vi "SaveDeviceHeader.vi"(0 "File Refnum in":refnum<file>, 2 "Channel Number":i32, 5 "Filename":string, 9 "Array Titles":string, 11 "error in (no error)":errorcluster, 12 "Temperature":dbl, 13 "Humidity":dbl, 14 "Strip Segment":string) -> (4 "File Refnum out":refnum<file>, 6 "Header string":string, 10 "error out":errorcluster)   [LabVIEW 2019]
uses:
  globals/QC_MeasurementSetup.vi
  globals/QC_RunInformation.vi
  <vilib>/regexp/Match Regular Expression.xnode
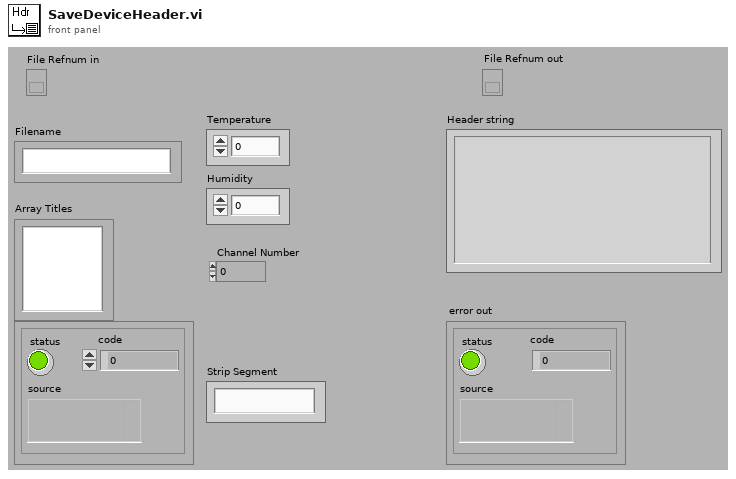
[diagram p1: front panel]
types:
  T1 = cluster{"User":string, " Institute":string, " Test Time":string, " Test Date":string, "Instruments":string, "Sensor IDS":string[], "IV Test?":bool, "CV Test? ":bool, "LCS Test? ":bool, "No. of Ch.":u16, " Current Sensor":string, " Current Test":string, "Arduino DP Map":string[], "Sensor BW":string[], "Sensor Types":string[], "Data directory":string, "7036 Channel Map":string[], "7054 1 Map":string[], "7054 2 Map ":string[], "7054 3 Map ":string[]}
  T2 = cluster{"Supply":refnum<class "SupplyControl.lvclass">, "LCR":refnum<class "LCRControl.lvclass">, "Arduino":refnum<class "ArduinoControl.lvclass">, "Switching":refnum<class "Switching.lvclass">, "SMU Name":string, " LCR Name":string, " Volt Name ":string, " Switching GPIB Address ":string, "Temperature Readout":enum16{"Read Arduino", "Enter manually"}, "Voltmeter Visa":refnum<visa-resource-name>}
  T3 = cluster{"Supply":refnum<class "SupplyControl.lvclass">, "LCR":refnum<class "LCRControl.lvclass">, "Initial Voltage [V]":dbl, "Final Voltage [V]":dbl, "Step Size [V]":dbl, "Step Interval [s]":i32, "Number Of Steps":u32, "AC frequency [Hz]":i32, "RC Configuration":u16, "AC amplitude [V]":dbl, "Ramp down steps [V]":dbl, "Ramp down Interval [s]":i32, "Set Current Limit?":bool, "Current Limit [µA]":dbl, "Temperature Readout":enum16{"Read Arduino", "Enter manually"}, "Arduino":refnum<class "ArduinoControl.lvclass">, "Supply Name":string, "LCR Name":string, "V_depletion Limit [V]":dbl, "Switching":refnum<class "Switching.lvclass">, "Matrix used?":bool, "Matrix X Channels":cluster{"Bias Supply / SMU LO":i32, "Bias Supply / SMU HI":i32, "CV Box LO":i32, "CV Box HI":i32, "CV Box LO IN":i32, "CV Box HI IN":i32, "Volt meter LO":i32, "Volt meter HI":i32, "Mux1 C1":i32, "Mux1 C2":i32, "Mux2 C1":i32, "Mux2 C2":i32}, "CV Test?":bool}
  T4 = cluster{"Bias Supply":refnum<class "SupplyControl.lvclass">, "SMU":refnum<class "SupplyControl.lvclass">, "LCR":refnum<class "LCRControl.lvclass">, "Probe Card Channels":i32, "Bias Voltage [V]":dbl, "First strip":i32, "Last strip":i32, "Base Voltage [V]":dbl, "Base Ramp Step [V]":dbl, "Base Ramp Interval [ms]":u32, "High Voltage [V]":dbl, "High Ramp Step [V]":dbl, "High Ramp Interval [ms]":u32, "AC frequency [Hz]":i32, "AC amplitude [V]":dbl, "RC Configuration":u16, "Single Needle":bool, "Temperature Readout":enum16{"Read Arduino", "Enter manually"}, "Arduino":refnum<class "ArduinoControl.lvclass">, "Fraction of good strips [%]":dbl, "ProbeStation":refnum<class "ProbeStationControl.lvclass">, "Switching":refnum<class "Switching.lvclass">, "Matrix used?":bool, "Matrix X Channels":cluster{"Bias Supply / SMU LO":i32, "Bias Supply / SMU HI":i32, "CV Box LO":i32, "CV Box HI":i32, "CV Box LO IN":i32, "CV Box HI IN":i32, "Volt meter LO":i32, "Volt meter HI":i32, "Mux1 C1":i32, "Mux1 C2":i32, "Mux2 C1":i32, "Mux2 C2":i32}, "Pinholes Y/N":bool, "Capacitance Y/N":bool, "Resistance Y/N":bool, "Bias Supply Name":string, "SMU Name":string, "LCR Name":string}
  T5 = cluster{"Sensor Serial No.:":string, "Wafer Serial No.:":string, "Batch:":string, "Manufacturer:":string, "Device Category:":string, "Database Serial No.:":string, "Date Initiated:":string, "Time Initiated:":string, "Test":string, "Instruments used:":string, "Probeplan used:":string, "End of Run comment:":string, "User:":string}
  T6 = cluster{"Supply":refnum<class "SupplyControl.lvclass">, "LCR":refnum<class "LCRControl.lvclass">, "Initial Voltage [V]":dbl, "Final Voltage [V]":dbl, "Step Size [V]":dbl, "Step Interval [s]":i32, "Number Of Steps":u32, "AC frequency [Hz]":i32, "RC Configuration":u16, "AC amplitude [V]":dbl, "Ramp down steps [V]":dbl, "Ramp down Interval [s]":i32, "Set Current Limit?":bool, "Current Limit [µA]":dbl, "Temperature Readout":enum16{"Read Arduino", "Enter manually"}, "Arduino":refnum<class "ArduinoControl.lvclass">, "Supply Name":string, "LCR Name":string, "C_is Limit [pF/cm]":dbl, "Switching":refnum<class "Switching.lvclass">, "Matrix used?":bool, "Matrix X Channels":cluster{"Bias Supply / SMU LO":i32, "Bias Supply / SMU HI":i32, "CV Box LO":i32, "CV Box HI":i32, "CV Box LO IN":i32, "CV Box HI IN":i32, "Volt meter LO":i32, "Volt meter HI":i32, "Mux1 C1":i32, "Mux1 C2":i32, "Mux2 C1":i32, "Mux2 C2":i32}}
  T7 = cluster{"Supply":refnum<class "SupplyControl.lvclass">, "Voltage [V]":dbl, "Measurement Interval [s]":i32, "Test Duration":u32, "Ramp up steps [V]":dbl, "Ramp up Interval [s]":u32, "Ramp down steps [V]":dbl, "Ramp down Interval [s]":i32, "Set Current Limit?":bool, "Current Limit [µA]":dbl, "Temperature Readout":enum16{"Read Arduino", "Enter manually"}, "Arduino":refnum<class "ArduinoControl.lvclass">, "Supply Name":string, "Maximum current fluctuation [%]":dbl, "Switching.lvclass":refnum<class "Switching.lvclass">, "Matrix used?":bool, "Matrix X Channels":cluster{"Bias Supply / SMU LO":i32, "Bias Supply / SMU HI":i32, "CV Box LO":i32, "CV Box HI":i32, "CV Box LO IN":i32, "CV Box HI IN":i32, "Volt meter LO":i32, "Volt meter HI":i32, "Mux1 C1":i32, "Mux1 C2":i32, "Mux2 C1":i32, "Mux2 C2":i32}, "LCS Test?":bool, "Number of Steps":i32, "Norm. to Temp.":dbl}
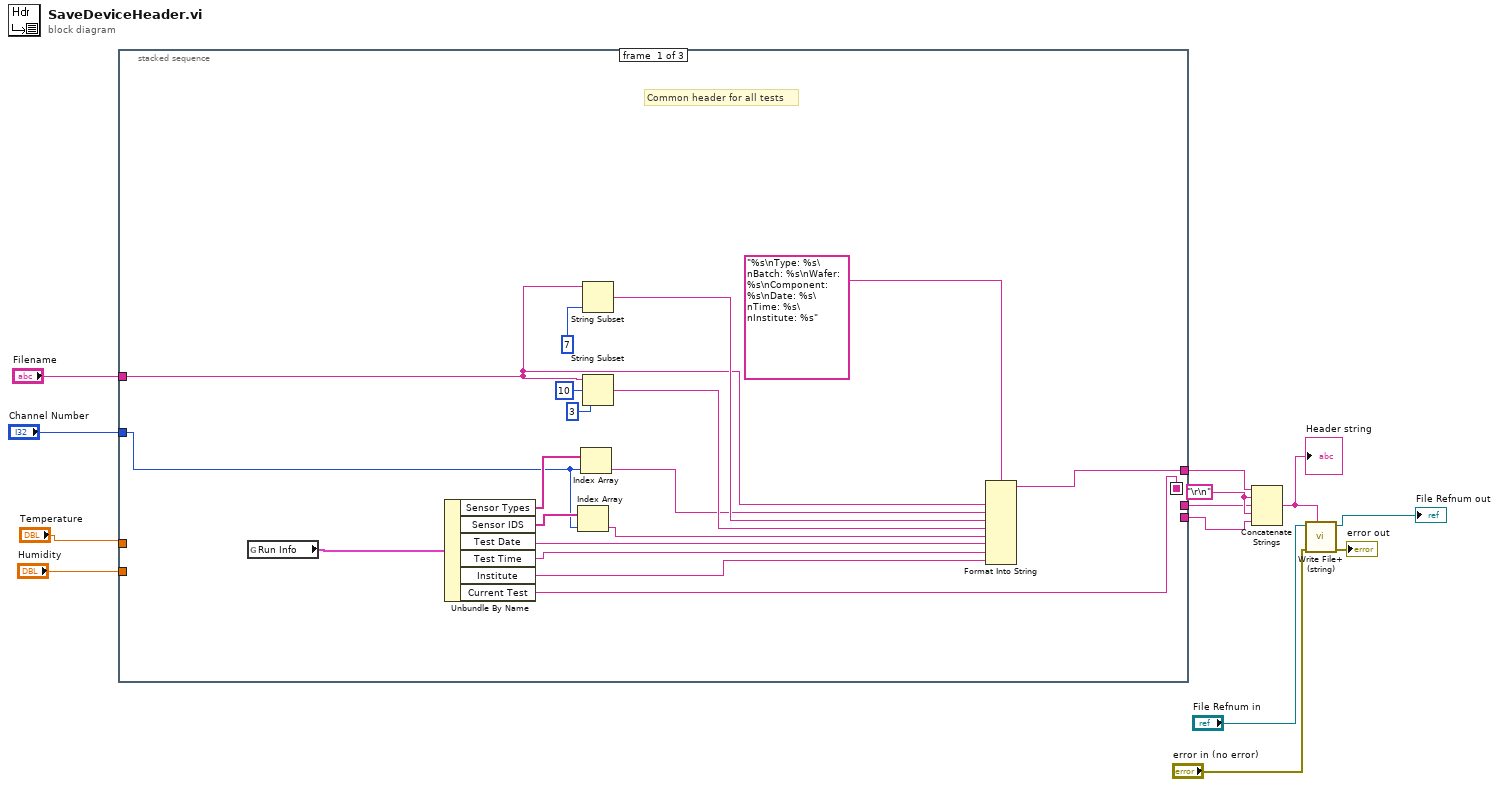
[diagram p0: block diagram]
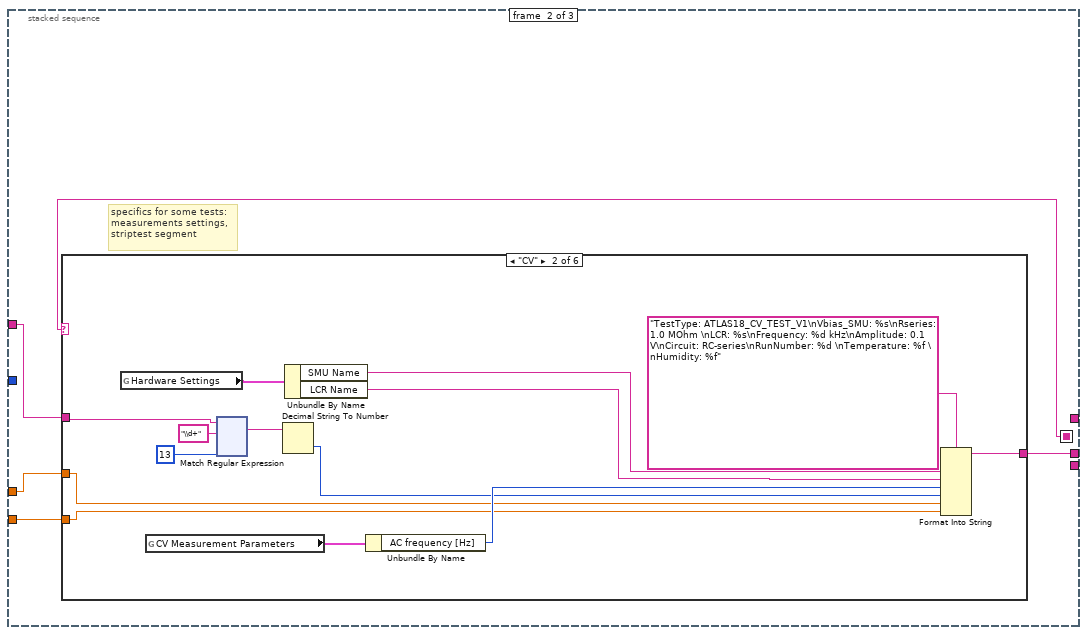
[diagram p2: hidden frame]
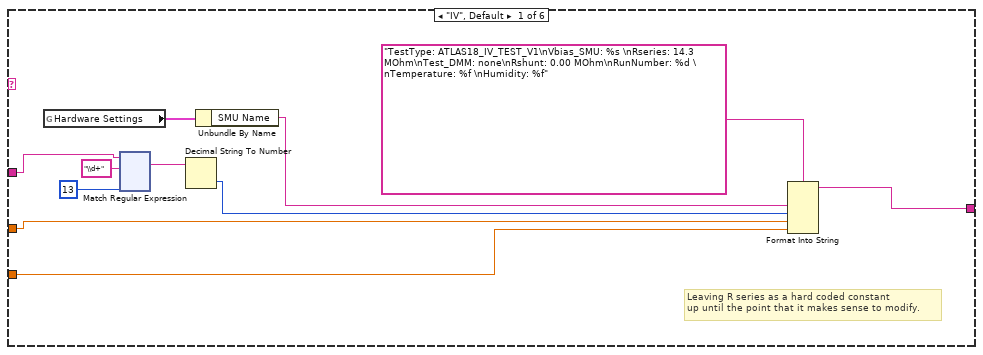
[diagram p3: hidden frame]
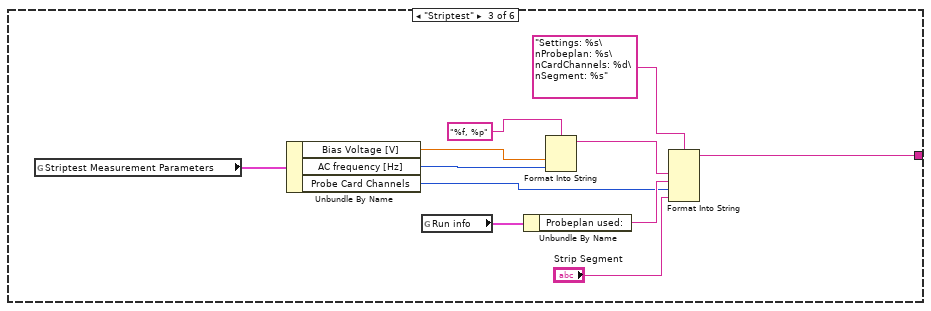
[diagram p4: hidden frame]
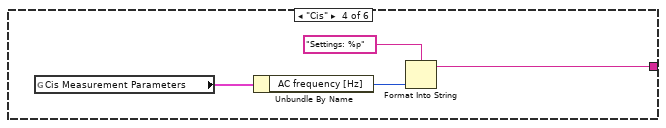
[diagram p5: hidden frame]
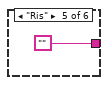
[diagram p6: hidden frame]
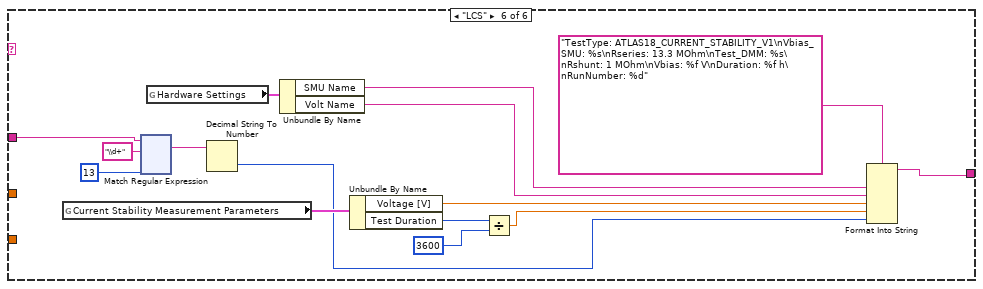
[diagram p7: hidden frame]
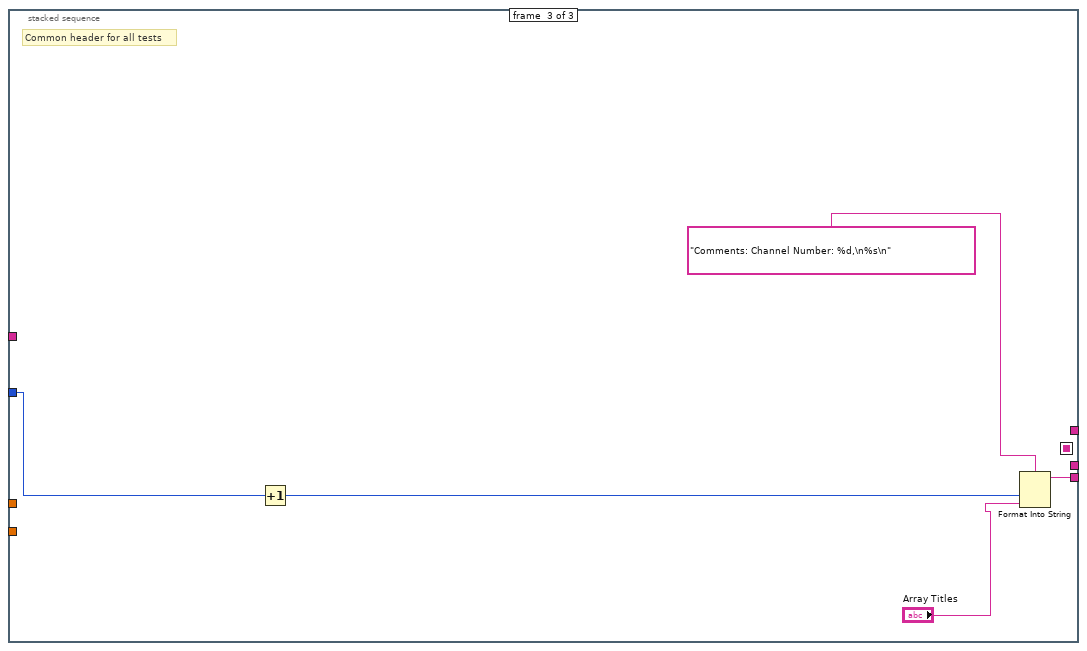
[diagram p8: hidden frame]
diagram:
  w9 = "\r\n"
  n1 = stacked-sequence {
    seq-local: [w15 _ _] -> [_ w36 _]
    tunnel: [_ w35 _] -> w8
    tunnel: [_ _ w438] -> w7
    tunnel: [w31 _ _] -> w6
    tunnel: "Channel Number" -> [w20 _ w437]
    tunnel: "Temperature" -> [_ w34 _]
    tunnel: "Humidity" -> [_ w33 _]
    tunnel: "Filename" -> [w14 w32 _]
    frame #0 {
      # "Common header for all tests"
      n2 = global read "QC_MeasurementSetup.vi" "Run Info"() -> (w22:T1)
      n3 = Unbundle By Name(w22) -> ("Sensor Types"=w24:string[], "Sensor IDS"=w21:string[], "Test Date"=w18:string, "Test Time"=w17:string, "Institute"=w16:string, "Current Test"=w15:string)
      n4 = Index Array(array=w21, index=w20) -> (element=w19:string)
      n5 = Index Array(array=w24, index=w20) -> (element=w23:string)
      n6 = String Subset(string=w14, length (rest)=7 ("length (rest)")) -> (substring=w25:string)  [unwired: 1 in]
      n7 = String Subset(string=w14, offset (0)=10, length (rest)=3 ("length (rest)")) -> (substring=w26:string)
      n8 = Format Into String(format string="%s\nType: %s\nBatch: %s\nWafer: %s\nComponent: %s\nDate: %s\nTime: %s\nInstitute: %s", w14, w23, w25, w26, w19, w18, w17, w16) -> (resulting string=w31:string)  [unwired: 2 in, 1 out]
    }
    frame #1 {
      # "specifics for some tests:\nmeasurements settings,\nstriptest segment"
      n9 = case shown="\"CV\"" w36 {
        tunnel: [w37 w173 w291 w301 "" w314] -> w35
        tunnel: w34 -> [w39 w163 _ _ _ _]
        tunnel: w33 -> [w38 w162 _ _ _ _]
        tunnel: w32 -> [w43 w169 _ _ _ w317]
        frame "IV", Default {
          # "Leaving R series as a hard coded constant\nup until the point that it makes sense to modify."
          n10 = global read "QC_MeasurementSetup.vi" "Hardware Settings"() -> (w42:T2)
          n11 = xnode "Match Regular Expression"("input string"=w43, "regular expression"="\\d+", "offset (0)"=u32 13 ("initial scan location")) -> ("whole match"=w44:string)  [unwired: 3 in, 4 out]
          n12 = Decimal String To Number(string=w44) -> (number=w40:i32)  [unwired: 2 in, 1 out]
          n13 = Unbundle By Name(w42) -> ("SMU Name"=w41:string)
          n14 = Format Into String(format string="TestType: ATLAS18_IV_TEST_V1\nVbias_SMU: %s \nRseries: 14.3 MOhm\nTest_DMM: none\nRshunt: 0.00 MOhm\nRunNumber: %d \nTemperature: %f \nHumidity: %f", w41, w40, w39, w38) -> (resulting string=w37:string)  [unwired: 2 in, 1 out]
        }
        frame "CV" {
          n15 = global read "QC_MeasurementSetup.vi" "Hardware Settings"() -> (w168:T2)
          n16 = global read "QC_MeasurementSetup.vi" "CV Measurement Parameters"() -> (w174:T3)
          n17 = xnode "Match Regular Expression"("input string"=w169, "regular expression"="\\d+", "offset (0)"=u32 13 ("initial scan location")) -> ("whole match"=w170:string)  [unwired: 3 in, 4 out]
          n18 = Decimal String To Number(string=w170) -> (number=w164:i32)  [unwired: 2 in, 1 out]
          n19 = Unbundle By Name(w168) -> ("SMU Name"=w167:string, "LCR Name"=w166:string)
          n20 = Unbundle By Name(w174) -> ("AC frequency [Hz]"=w165:i32)
          n21 = Format Into String(format string="TestType: ATLAS18_CV_TEST_V1\nVbias_SMU: %s\nRseries: 1.0 MOhm \nLCR: %s\nFrequency: %d kHz\nAmplitude: 0.1 V\nCircuit: RC-series\nRunNumber: %d \nTemperature: %f \nHumidity: %f", w167, w166, w165, w164, w163, w162) -> (resulting string=w173:string)  [unwired: 2 in, 1 out]
        }
        frame "Striptest" {
          n22 = global read "QC_MeasurementSetup.vi" "Striptest Measurement Parameters"() -> (w299:T4)
          n23 = Unbundle By Name(w299) -> ("Bias Voltage [V]"=w296:dbl, "AC frequency [Hz]"=w295:i32, "Probe Card Channels"=w292:i32)
          n24 = global read "QC_RunInformation.vi" "Run info"() -> (w300:T5)
          n25 = Unbundle By Name(w300) -> ("Probeplan used:"=w293:string)
          n26 = Format Into String(format string="%f, %p", w296, w295) -> (resulting string=w294:string)  [unwired: 2 in, 1 out]
          n27 = Format Into String(format string="Settings: %s\nProbeplan: %s\nCardChannels: %d\nSegment: %s", w294, w293, w292, "Strip Segment") -> (resulting string=w291:string)  [unwired: 2 in, 1 out]
        }
        frame "Cis" {
          n28 = global read "QC_MeasurementSetup.vi" "Cis Measurement Parameters"() -> (w302:T6)
          n29 = Unbundle By Name(w302) -> ("AC frequency [Hz]"=w304:i32)
          n30 = Format Into String(format string="Settings: %p", w304) -> (resulting string=w301:string)  [unwired: 2 in, 1 out]
        }
        frame "Ris" {
        }
        frame "LCS" {
          n31 = global read "QC_MeasurementSetup.vi" "Current Stability Measurement Parameters"() -> (w312:T7)
          n32 = xnode "Match Regular Expression"("input string"=w317, "regular expression"="\\d+", "offset (0)"=u32 13 ("initial scan location")) -> ("whole match"=w318:string)  [unwired: 3 in, 4 out]
          n33 = global read "QC_MeasurementSetup.vi" "Hardware Settings"() -> (w315:T2)
          n34 = Decimal String To Number(string=w318) -> (number=w307:i32)  [unwired: 2 in, 1 out]
          n35 = Unbundle By Name(w315) -> ("SMU Name"=w313:string, "Volt Name"=w306:string)
          n36 = Unbundle By Name(w312) -> ("Voltage [V]"=w311:dbl, "Test Duration"=w310:u32)
          n37 = Divide(x=w310, y=u32 3600) -> (x/y=w308:dbl)
          n38 = Format Into String(format string="TestType: ATLAS18_CURRENT_STABILITY_V1\nVbias_SMU: %s\nRseries: 13.3 MOhm\nTest_DMM: %s\nRshunt: 1 MOhm\nVbias: %f V\nDuration: %f h\nRunNumber: %d", w313, w306, w311, w308, w307) -> (resulting string=w314:string)  [unwired: 2 in, 1 out]
        }
      }
    }
    frame #2 {
      # "Common header for all tests"
      n39 = Increment(x=w437) -> (x+1=w436:i32)
      n40 = Format Into String(format string="Comments: Channel Number: %d,\n%s\n", w436, "Array Titles") -> (resulting string=w438:string)  [unwired: 2 in, 1 out]
    }
  }
  n41 = Concatenate Strings(w6, w9, w8, w9, w7) -> (w5:string)
  "Header string" <- w5
  n42 = call <vilib>:"Write File+ (string).vi"("string"=w5, "error in (no error)"="error in (no error)", "refnum"="File Refnum in") -> ("error out"=→"error out":errorcluster, "dup refnum"=→"File Refnum out":refnum<file>)  [unwired: 4 in, 1 out]
